vi "Host Buffers Status.vi"(4 "output.Reset":bool, 6 "input.Reset":bool, 8 "output.Empty Elements Remaining":u32, 9 "output.Elements In Region":u32, 10 "input.Elements Remaining":u32, 11 "input.Elements In Region":u32) -> (0 "output.Host Buffer Status":cluster{u32, u32, u32}, 1 "output.Samples Written":u64 caption="Samples Written", 2 "input.Host Buffer Status":cluster{u32, u32, u32}, 3 "input.Samples Read":u64 caption="Samples Read")   [LabVIEW 2016]
doc: "This SubVI Monitors the Host Side Buffers for both DMA FIFOs. It returns the number of samples read from and written to the FIFOs as well as the current status of the Host Side Buffers."
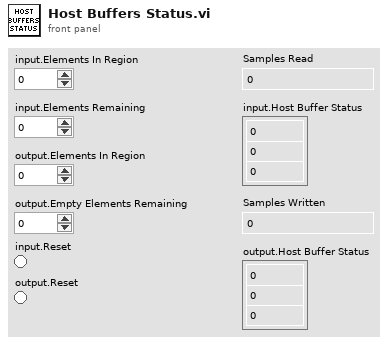
[diagram p1: front panel]
types:
  T1 = cluster{u32, "input.Elements Remaining":u32, "Running Max":u32}
  T2 = cluster{u32, "output.Empty Elements Remaining":u32, "Running Max":u32}
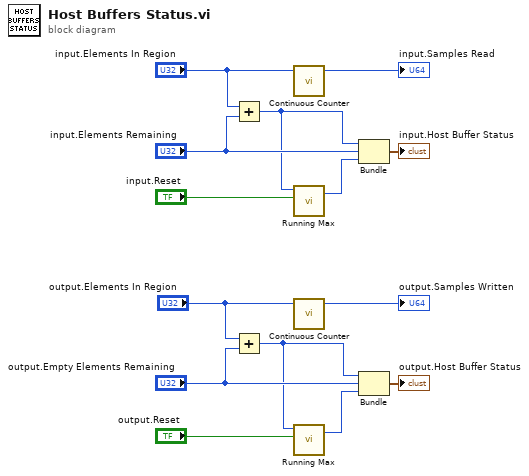
[diagram p0: block diagram]
diagram:
  n1 = Add(x="input.Elements In Region", y="input.Elements Remaining") -> (x+y=w10:u32)
  n2 = Add(x="output.Elements In Region", y="output.Empty Elements Remaining") -> (x+y=w4:u32)
  n3 = call "Continuous Counter.vi"("value"="input.Elements In Region") -> ("count"=→"input.Samples Read":u64)  [unwired: 6 in]
  n4 = call "Running Max.vi"("Reset"="input.Reset", "Next Value"=w10) -> ("Running Max"=w9:u32)  [unwired: 5 in]
  n5 = call "Continuous Counter.vi"("value"="output.Elements In Region") -> ("count"=→"output.Samples Written":u64)  [unwired: 6 in]
  n6 = call "Running Max.vi"("Reset"="output.Reset", "Next Value"=w4) -> ("Running Max"=w14:u32)  [unwired: 5 in]
  n7 = Bundle(w10, "input.Elements Remaining"="input.Elements Remaining", "Running Max"=w9) -> (→"input.Host Buffer Status":T1)  [unwired: 1 in]
  n8 = Bundle(w4, "output.Empty Elements Remaining"="output.Empty Elements Remaining", "Running Max"=w14) -> (→"output.Host Buffer Status":T2)  [unwired: 1 in]
